vi "Configure Curve Header.vi"(0 "VISA resource name":refnum<visa-resource-name>, 1 "Curve Data Format (1:mV/K)":u16(ring)=1 items=["mV/K"=1, "V/K"=2, "Ohms/K"=3, "Log Ohms/K"=4], 2 "Limit Value (375.000)":dbl=375.0 format="%.3f", 5 "Curve (21)":dbl=21.0, 7 "Curve Name (\"\")":string, 9 "Curve Serial Number (\"\")":string, 11 "error in (no error)":errorcluster, 12 "Coefficient (1:Negative)":u16(ring)=1 items=["Negative"=1, "Positive"=2]) -> (4 "VISA resource name out":refnum<visa-resource-name>, 15 "error out":errorcluster)   [LabVIEW 2010, in "Lake Shore 350.lvlib"]
doc: "Configures a curve header. Each curve has parameters that are used for identification and to allow the instrument to use the curve effectively. The parameters must be set correctly before a curve can be used for temperature conversion or tempersture control."
uses:
  <instrlib>/Lake Shore 350/Lake Shore 350.lvlib
  Instance           1 30Saved   Configure Curve Header .vi
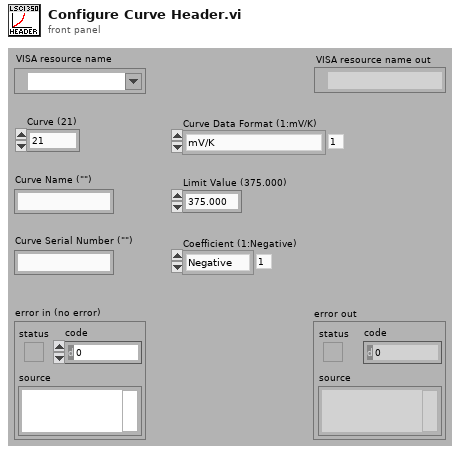
[diagram p1: front panel]
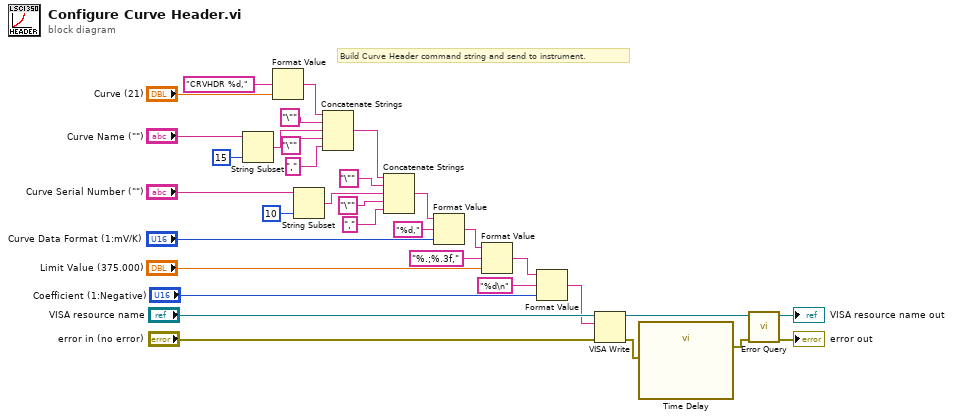
[diagram p0: block diagram]
diagram:
  # "Build Curve Header command string and send to instrument."
  n1 = String Subset(string="Curve Name (\"\")", length (rest)=15) -> (substring=w8:string)  [unwired: 1 in]
  n2 = Format Value(format string="CRVHDR %d,", value (0)="Curve (21)") -> (output string=w22:string)  [unwired: 1 in]
  n3 = String Subset(string="Curve Serial Number (\"\")", length (rest)=10) -> (substring=w3:string)  [unwired: 1 in]
  n4 = Concatenate Strings(w22, "\"", w8, "\"", ",") -> (w4:string)
  n5 = Concatenate Strings(w4, "\"", w3, "\"", ",") -> (w18:string)
  n6 = Format Value(string ("")=w18, format string="%d,", value (0)="Curve Data Format (1:mV/K)") -> (output string=w17:string)
  n7 = Format Value(string ("")=w17, format string="%.;%.3f,", value (0)="Limit Value (375.000)") -> (output string=w13:string)
  n8 = Format Value(string ("")=w13, format string="%d\n", value (0)="Coefficient (1:Negative)") -> (output string=w11:string)
  n9 = VISA Write(VISA resource name="VISA resource name", write buffer=w11, error in (no error)="error in (no error)") -> (VISA resource name out=w30:refnum<visa-resource-name>, error out=w16:errorcluster)  [unwired: 1 out]
  n10 = call "Time Delay"("error in (no error)"=w16) -> ("error out"=w15:errorcluster)  [unwired: 10 in]
  n11 = call <instrlib>:"Error Query.vi"("error in (no error)"=w15, "VISA resource name"=w30) -> ("error out"=→"error out":errorcluster, "VISA resource name out"=→"VISA resource name out":refnum<visa-resource-name>)  [unwired: 7 in, 1 out]
